vi "SetMeasFuncList.vi"(8 "error in (no error)":errorcluster caption="entrée d'erreur (pas d'erreur)", 10 "ListRef":refnum<vi>, 11 "Experiment en entrée":refnum<class "Experiment.lvclass"> caption="DNL_LabVIEW Object in") -> (0 "error out":errorcluster caption="sortie d'erreur", 3 "Experiment en sortie":refnum<class "Experiment.lvclass"> caption="DNL_LabVIEW Object out")   [LabVIEW 2019, in "Experiment.lvclass"]
uses:
  Experiment.lvclass
  Experiment.lvclass/Experiment.ctl
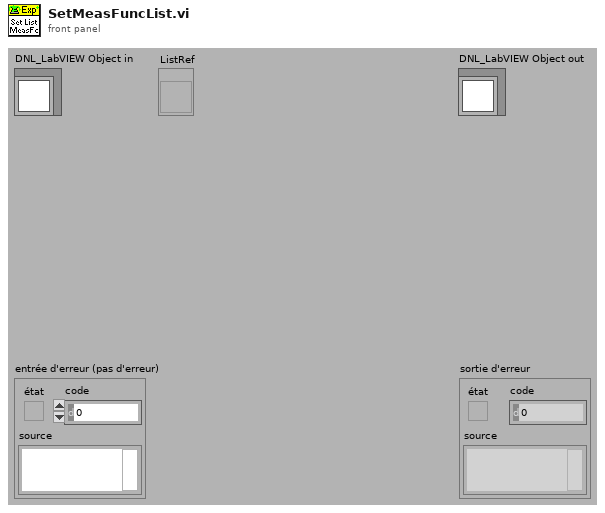
[diagram p1: front panel]
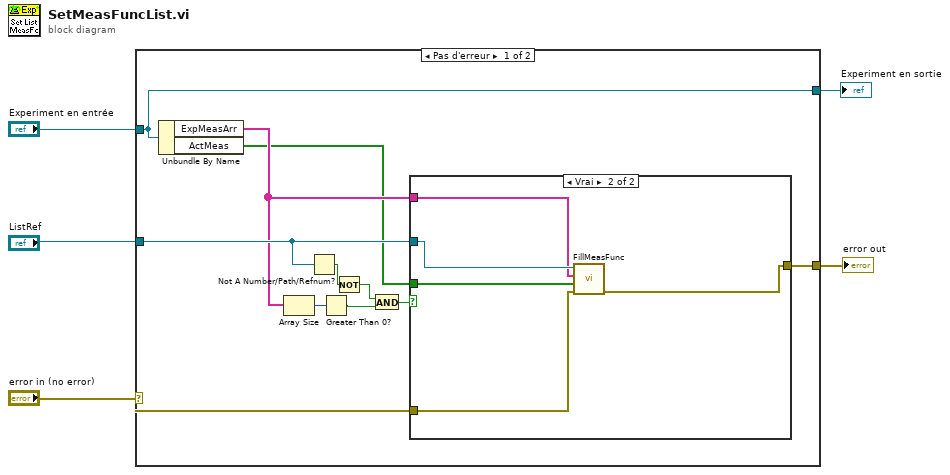
[diagram p0: block diagram]
diagram:
  n1 = case shown="Pas d'erreur" "error in (no error)" {
    selector: "error in (no error)" -> [w7 w24]
    tunnel: [w16 w24] -> w4
    tunnel: [w8 w23] -> w2
    tunnel: "Experiment en entrée" -> [w8 w23]
    tunnel: "ListRef" -> [w13 _]
    frame No Error {
      n2 = Unbundle By Name(w8) -> ("ExpMeasArr"=w11:string[], "ActMeas"=w6:bool[])
      n3 = Array Size(array=w11) -> (size(s)=w10:i32)
      n4 = Not A Number/Path/Refnum?(number/path/refnum=w13) -> (NaN/Path/Refnum?=w14:bool)
      n5 = Greater Than 0?(x=w10) -> (x > 0?=w9:bool)
      n6 = Not(x=w14) -> (.not. x?=w12:bool)
      n7 = And(x=w12, y=w9) -> (x .and. y?=w15:bool)
      n8 = case shown="Vrai" w15 {
        tunnel: w13 -> [_ w22]
        tunnel: w7 -> [w17 w19]
        tunnel: [w17 w18] -> w16
        tunnel: w11 -> [_ w21]
        tunnel: w6 -> [_ w20]
        frame False {
        }
        frame True {
          n9 = call "FillMeasFunc.vi"("ErrorIn(No Error)"=w19, "ActMeas"=w20, "MeasFunc"=w21, "ListRef"=w22) -> ("sortie d'erreur"=w18:errorcluster)  [unwired: 6 in, 1 out]
        }
      }
    }
    frame Error {
    }
  }
  "error out" <- w4
  "Experiment en sortie" <- w2
